vi "GetRS232.vi"(0 "VISA resource name":refnum<visa-resource-name>="COM5", 1 "Bytes To Read":i32=3, 2 "Control":refnum<vi>, 3 "Type":bool, 4 "Limit":i32) -> (5 "Data":string, 6 "error out":errorcluster)   [LabVIEW 2014]
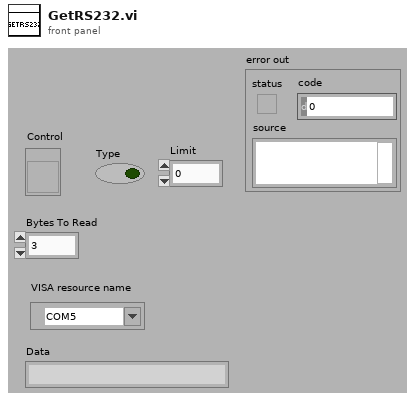
[diagram p1: front panel]
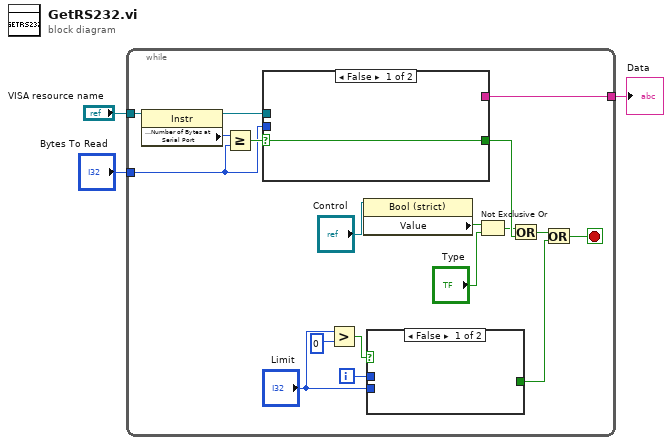
[diagram p0: block diagram]
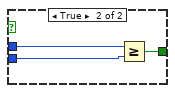
[diagram p2: hidden frame]
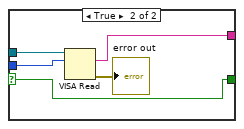
[diagram p3: hidden frame]
diagram:
  n1 = while {
    tunnel: [w21] -> w1
    tunnel: "VISA resource name" -> [w17]
    tunnel: "Bytes To Read" -> [w16]
    i -> [w6]
    stop <- w9 stop-if-true
    n2 = property class="Instr"(reference=w17) -> (reference out=w18:refnum<visa-resource-name>, "Serial Settings:Number of Bytes at Serial Port"=w20:u32)  [unwired: 1 in, 1 out]
    n3 = Greater Or Equal?(x=w20, y=w16) -> (x >= y?=w19:bool)
    n4 = case shown="False" w19 {
      selector: w19 -> [w25 w27]
      tunnel: [_ w30] -> w21
      tunnel: w16 -> [_ w29]
      tunnel: w18 -> [_ w28]
      tunnel: [w25 w27] -> w14
      frame False {
      }
      frame True {
        n5 = VISA Read(VISA resource name=w28, byte count=w29) -> (read buffer=w30:string, error out=→"error out":errorcluster)  [unwired: 1 in, 2 out]
      }
    }
    n6 = Greater?(x="Limit", y=0) -> (0:w7:bool)
    n7 = property class="Bool (strict)"(reference="Control") -> ("Value"=w13:bool)  [unwired: 1 in, 2 out]
    n8 = case shown="False" w7 {
      tunnel: w6 -> [_ w24]
      tunnel: "Limit" -> [_ w23]
      tunnel: [_ w22] -> w4
      frame False {
      }
      frame True {
        n9 = Greater Or Equal?(x=w24, y=w23) -> (x >= y?=w22:bool)
      }
    }
    n10 = Not Exclusive Or(1:"Type", 2:w13) -> (0:w12:bool)
    n11 = Or(x=w12, y=w14) -> (x .or. y?=w10:bool)
    n12 = Or(x=w10, y=w4) -> (x .or. y?=w9:bool)
  }
  "Data" <- w1
